vi "CheckBandejas.vi"() -> ()   [LabVIEW 2019]
uses:
  TYPE'S DEF/INPUT_TRASPASO_ASICS.ctl
panel:
  in  "TRASPASO ASICS INPUT":T1={"COORD X ORIGEN"=0, "COORD  Y ORIGEN"=0, "NºASICS A MOVER"=1, "BANDEJA ORIGEN"=enum."BANDEJA ENTRADA", "BANDEJA DESTINO"=enum."BANDEJA ENTRADA", "COORD X DESTINO "=0, "COORD  Y DESTINO "=0, "CONTEO TRASLADOS"=0}
  out "error out":errorcluster
  in  "error in (no error)":errorcluster
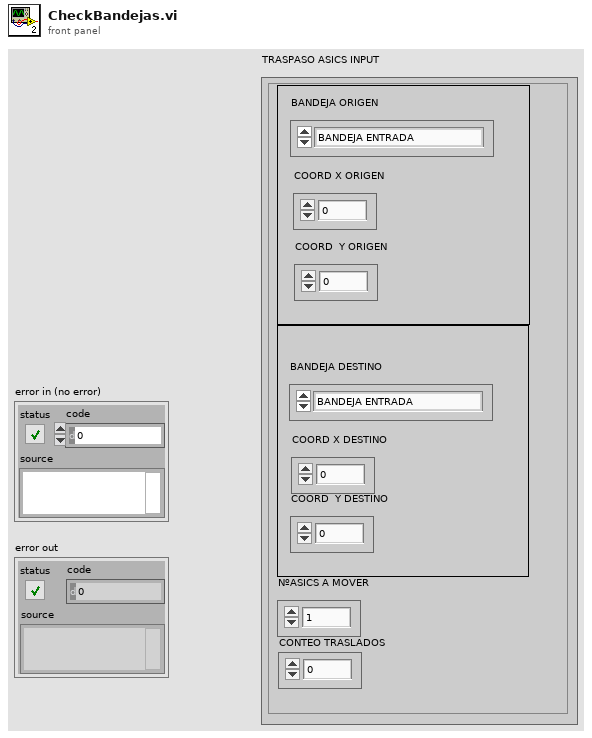
[diagram p1: front panel]
types:
  T1 = typedef "INPUT_TRASPASO_ASICS.ctl" = cluster{"COORD X ORIGEN":u16, "COORD  Y ORIGEN":u16, "NºASICS A MOVER":u32, "BANDEJA ORIGEN":enum16{"NINGUNA", "BANDEJA ENTRADA", "BANDEJA OK", "BANDEJA NOK"}, "BANDEJA DESTINO":enum16{"NINGUNA", "BANDEJA ENTRADA", "BANDEJA OK", "BANDEJA NOK"}, "COORD X DESTINO ":u16, "COORD  Y DESTINO ":u16, "CONTEO TRASLADOS":u32}
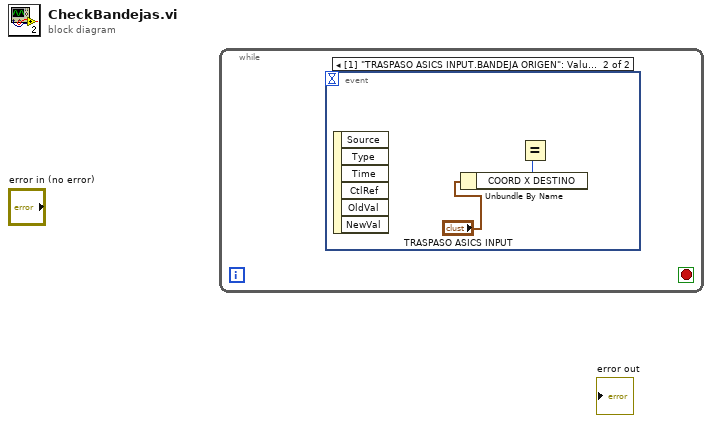
[diagram p0: block diagram]
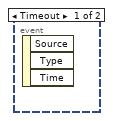
[diagram p2: hidden frame]
diagram:
  n1 = while {
    stop <- _ stop-if-true
    n2 = event shown="[1] \"TRASPASO ASICS INPUT.BANDEJA ORIGEN\": Value Change" {
      selector: _ -> [_ _]
      dyn-events: _ -> [_ _]
      timeout: _ -> [_ _]
      event Timeout {
        n3 = event-data() -> ()  [unwired: 1 in, 3 out]
      }
      event Value Change {
        n4 = event-data() -> ()  [unwired: 1 in, 6 out]
        n5 = Unbundle By Name("TRASPASO ASICS INPUT") -> ("COORD X DESTINO"=w2:u16)
        n6 = Equal?(y=w2) -> ()  [unwired: 1 in, 1 out]
      }
    }
  }
